vi "ResetDisplayChartDialog.vi"(8 "Error In":errorcluster, 11 "VI Ref In":refnum<vi>) -> (0 "Error Out":errorcluster, 3 "VI Ref Out":refnum<vi>)   [LabVIEW 2013]
uses:
  <vilib>/Utility/miscctls.llb/LVPointTypeDef.ctl
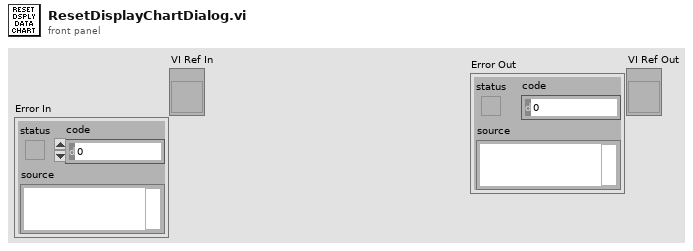
[diagram p1: front panel]
types:
  T1 = typedef "LVPointTypeDef.ctl" = cluster{"Horizontal":i16, "Vertical":i16}
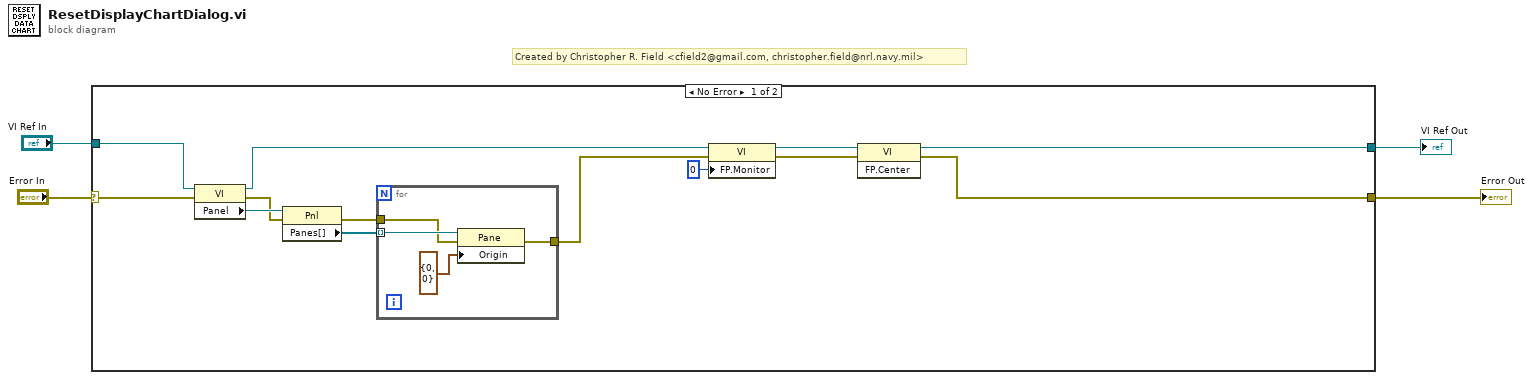
[diagram p0: block diagram]
diagram:
  # "Created by Christopher R. Field <cfield2@gmail.com, christopher.field@nrl.navy.mil>"
  n1 = case shown="No Error" "Error In" {
    selector: "Error In" -> [w13 w23]
    tunnel: [w5 w23] -> w4
    tunnel: "VI Ref In" -> [w12 w22]
    tunnel: [w6 w22] -> w1
    frame No Error {
      n2 = property class="VI"(reference=w12, error in=w13) -> (reference out=w11:refnum<vi>, error out=w16:errorcluster, "Panel"=w17:refnum<vi>)
      n3 = property class="Pnl"(reference=w17, error in=w16) -> (error out=w14:errorcluster, "Panes[]"=w15:refnum<vi>[])  [unwired: 1 out]
      n4 = for {
        tunnel: w15 -> [w21] mode=indexing
        tunnel: w14 -> [w19]
        tunnel: [w18] -> w10
        n5 = property class="Pane"(reference=w21, error in=w19, "Origin"=T1 {"Horizontal"=0, "Vertical"=0}) -> (error out=w18:errorcluster)  [unwired: 1 out]
      }
      n6 = property class="VI"(reference=w11, error in=w10, "FP.Monitor"=u16 0 ("Front Panel Window:Monitor")) -> (reference out=w8:refnum<vi>, error out=w7:errorcluster)
      n7 = invoke class="VI" method="FP.Center"(reference=w8, error in=w7) -> (reference out=w6:refnum<vi>, error out=w5:errorcluster)  [unwired: 1 in, 1 out]
    }
    frame Error {
    }
  }
  "Error Out" <- w4
  "VI Ref Out" <- w1
